vi "Shooter Controller.vi"(8 "error in":errorcluster) -> ()   [LabVIEW 2020]
doc: "This VI executes continuously carrying out the current operation and responding to updates or new operations. It will often contain the timing or control code that is difficult to place directly in TeleOp. This VI generally opens all sensors and motors and isolates the rest of the robot code from knowing how the operations are carried out."
uses:
  <vilib>/Rock Robotics/WPI/Framework/Completion Status.ctl
  Shooter Setpoints.ctl
  Shooter Operations.ctl
  <vilib>/Rock Robotics/WPI/SafetyOutput/WPI_SafetyOutputConfigMenu.ctl
  <vilib>/Rock Robotics/WPI/ThirdParty/REV Robotics/REVLib/Typedef/Spark MAX Motor Type.ctl
  <vilib>/Rock Robotics/WPI/ThirdParty/REV Robotics/REVLib/Typedef/Spark MAX Idle Mode.ctl
  <vilib>/Rock Robotics/Network Tables/NT Write Number.vi
panel:
  in  "Interactive Values":T1
  out "Current\nCmd":string
  in  "Buttons":cluster{"Execute Cmd":bool, "Abort Cmd":bool}
  out "Command Timing":cluster{"Start Time (ms)":u32, "Iterations":i32}
  out "Status":T3
  # "Tip: It may be helpful to observe inputs and sensor values.\nYou may also want to display tuning or debugging controls."
  # "Interactive Command: You may fill in the settings for a command\nand schedule it with the Execute button. You can observe and abort\nany command while fine tuning the code for the controller."
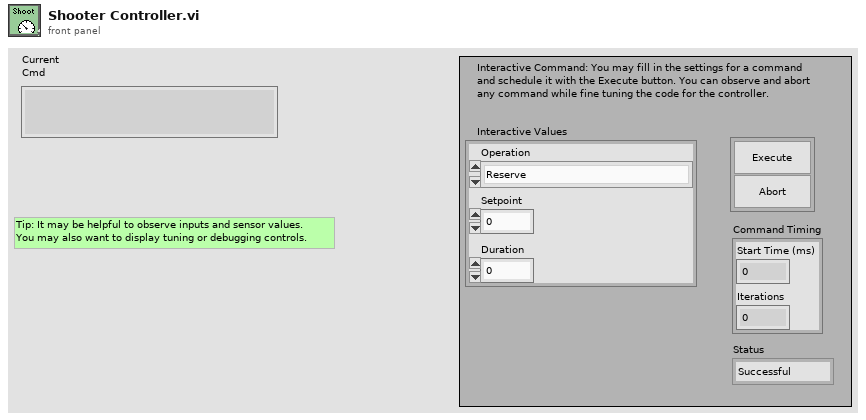
[diagram p1: front panel]
types:
  T1 = typedef "Shooter Setpoints.ctl" = cluster{"Operation":T2, "Setpoint":dbl, "Duration":dbl}
  T2 = typedef "Shooter Operations.ctl" = enum16{"Reserve", "Read Current", "Immediate", "For Time ", "Stop"}
  T3 = typedef "Completion Status.ctl" = enum16{"Successful", "Aborted", "Incomplete"}
  T4 = typedef "Spark MAX Idle Mode.ctl" = enum16{"Coast", "Brake"}
  T5 = typedef "Spark MAX Motor Type.ctl" = enum16{"Brushed", "Brushless"}
  T6 = typedef "WPI_SafetyOutputConfigMenu.ctl" = enum16{"Enable", "Disable"}
  T7 = typedef "WPI_MotorControlDeviceRef.ctl" = cluster{"DeviceStatus":errorcluster, "Type":T8, "PWM":cluster{"PWM Channel":T9, "DeadBand":T10}, "CAN":cluster{"Device Number":u8, "SetOutput VI Ref":variant, "GetOutput VI Ref":variant, "Enable VI Ref":variant, "Disable VI Ref":variant, "Data":variant}, "Invert":bool, "DIO PWM":cluster{"PWM \"Enable\" Channel":T9, "DIOChannel":T11, "PWM Rate":dbl}}
  T8 = typedef "WPI_MotorControlType.ctl" = enum16{"PWM", "CAN", "DIO PWM"}
  T9 = typedef "FPGA_DIOPWMChannel.ctl" = enum8{"PWM 0", "PWM 1", "PWM 2", "PWM 3", "PWM 4", "PWM 5", "PWM 6", "PWM 7", "PWM 8", "PWM 9", "PWM MXP 0", "PWM MXP 1", "PWM MXP 2", "PWM MXP 3", "PWM MXP 4", "PWM MXP 5", "PWM MXP 6", "PWM MXP 7", "PWM MXP 8", "PWM MXP 9", "Invalid"}
  T10 = typedef "WPI_PWMDeadband.ctl" = cluster{"Name":string, "maxPositivePwm":i32, "minPositivePwm":i32, "centerPwm":i32, "maxNegativePwm":i32, "minNegativePwm":i32, "angularRange":u16}
  T11 = typedef "FPGA_DIOChannel.ctl" = enum8{"DIO 0", "DIO 1", "DIO 2", "DIO 3", "DIO 4", "DIO 5", "DIO 6", "DIO 7", "DIO 8", "DIO 9", "DIO MXP 0", "DIO MXP 1", "DIO MXP 2", "DIO MXP 3", "DIO MXP 4", "DIO MXP 5", "DIO MXP 6", "DIO MXP 7", "DIO MXP 8", "DIO MXP 9", "DIO MXP 10", "DIO MXP 11", "DIO MXP 12", "DIO MXP 13", "DIO MXP 14", "DIO MXP 15", "SPI Port CS1", "SPI Port CS2", "SPI Port CS3", "SPI Port MISO", "SPI Port MOSI", "Invalid"}
  T12 = typedef "Command Status Info.ctl" = cluster{"Name":string, "Status":T3, "notifier out":T13}
  T13 = typedef "Completion Notifier.ctl" = refnum<notifier>
  T14 = cluster{"Current Command":T1, "Command Timing":cluster{"Start Time (ms)":u32, "Iterations":i32}, "Command Arguments":cluster{"Command Info":T12, "Description":string, "Default Command":T1, "queue out":refnum<queue>, "Subsystem Name":string}}
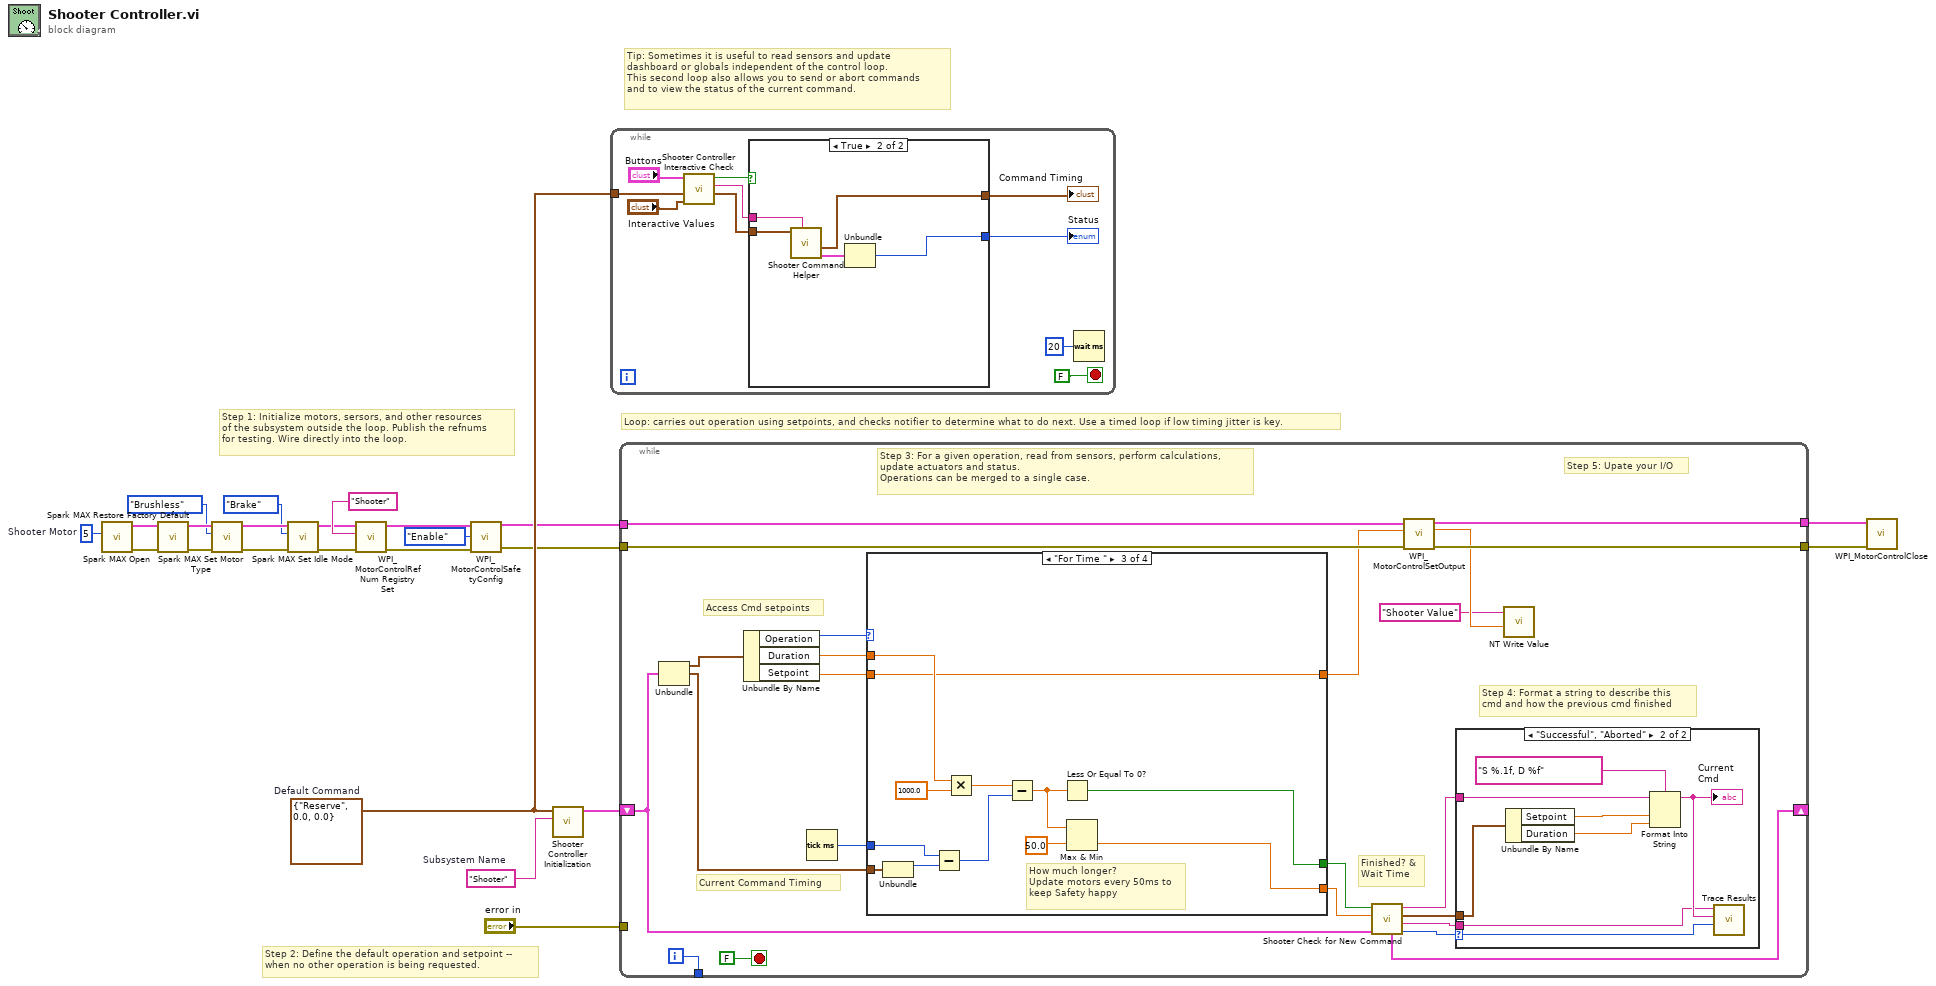
[diagram p0: block diagram]
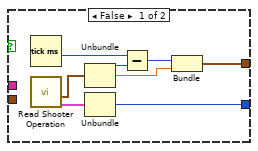
[diagram p2: hidden frame]
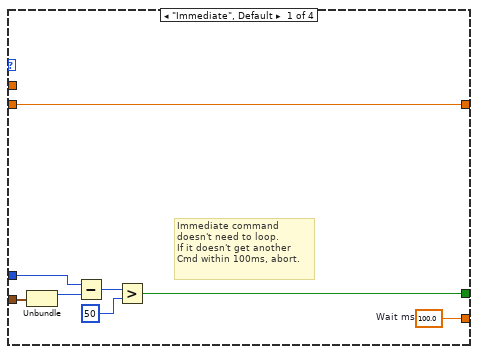
[diagram p4: hidden frame]
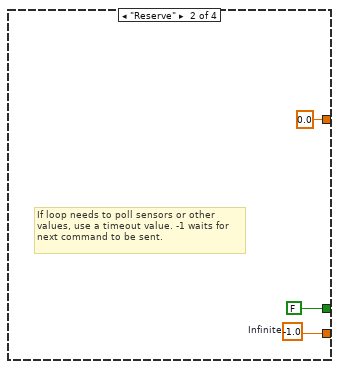
[diagram p5: hidden frame]
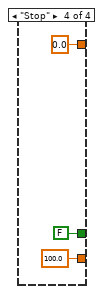
[diagram p6: hidden frame]
diagram:
  w1 = u8 5  # Shooter Motor
  w19 = T1 {"Operation"=enum."Reserve", "Setpoint"=0.0, "Duration"=0.0}  # Default Command
  w20 = "Shooter"  # Subsystem Name
  # "Tip: Sometimes it is useful to read sensors and update\ndashboard or globals independent of the control loop.\nThis second loop also allows you to send or abort commands\nand to view the status of the current command."
  # "Step 2: Define the default operation and setpoint --\nwhen no other operation is being requested."
  # "Step 1: Initialize motors, sersors, and other resources\nof the subsystem outside the loop. Publish the refnums\nfor testing. Wire directly into the loop."
  # "Loop: carries out operation using setpoints, and checks notifier to determine what to do next. Use a timed loop if low timing jitter is key."
  n1 = call <vilib>:"Spark MAX Open.vi"("Device Number"=w1) -> ("error out"=w18:errorcluster, "MotorControlDeviceRef"=w17:T7)  [unwired: 9 in]
  n2 = call <vilib>:"Spark MAX Restore Factory Default.vi"("error in"=w18, "MotorControlDeviceRef"=w17) -> ("error out"=w16:errorcluster, "MotorControlDeviceRef"=w15:T7)  [unwired: 8 in]
  n3 = call <vilib>:"Spark MAX Set Motor Type.vi"("error in (no error)"=w16, "Motor Type"=Spark_MAX_Motor_Type."Brushless", "MotorControlDevRef"=w15) -> ("error out"=w14:errorcluster, "MotorControlDeviceRef"=w13:T7)  [unwired: 7 in]
  n4 = call <vilib>:"Spark MAX Set Idle Mode.vi"("Idle Mode"=Spark_MAX_Idle_Mode."Brake", "MotorControlDeviceRef in"=w13) -> ("MotorControlDeviceRef out"=w7:T7)  [unwired: 8 in, 1 out]
  n5 = call <vilib>:"WPI_MotorControlRefNum Registry Set.vi"("error in (no error)"=w14, "refnum name"="Shooter", "MotorControlDevRef"=w7) -> ("error out"=w10:errorcluster, "MotorControlDevRef"=w12:T7)  [unwired: 7 in]
  n6 = call <vilib>:"WPI_MotorControlSafetyConfig.vi"("error in (no error)"=w10, "mode"=WPI_SafetyOutputConfigMenu."Enable", "MotorControlDevRef"=w12) -> ("error out"=w2:errorcluster, "MotorControlDevRef"=w5:T7)  [unwired: 7 in]
  n7 = call "Shooter Controller Initialization.vi"("Subsystem Name"=w20, "Default Command"=w19) -> ("Current Command"=w21:T14)  [unwired: 9 in]
  n8 = while {
    tunnel: w19 -> [w29]
    stop <- FALSE stop-if-true
    n9 = call "Shooter Controller Interactive Check.vi"("Interactive Command in"="Interactive Values", "Default Command"=w29, "Buttons"="Buttons") -> ("Interactive Command out"=w26:T1, "Trace String"=w27:string, "Schedule"=w28:bool)  [unwired: 6 in]
    n10 = case shown="True" w28 {
      tunnel: [w40 w45] -> w25
      tunnel: w26 -> [_ w43]
      tunnel: [w36 w41] -> w24
      tunnel: w27 -> [_ w44]
      frame False {
        n11 = Tick Count (ms)() -> (millisecond timer value=w35:u32)
        n12 = call "Read Shooter Operation.vi"() -> ("Command Info"=w33:T12, "SubSystem Data"=w34:T1)  [unwired: 9 in, 1 out]
        n13 = Unbundle(w34) -> ("Operation"=w39:T2, "Setpoint"=w37:dbl)  [unwired: 1 out]
        n14 = Unbundle(w33) -> ("Status"=w40:T3)  [unwired: 2 out]
        n15 = Subtract(x=w35, y=w39) -> (x-y=w38:u32)
        n16 = Bundle(w38, "Setpoint"=w37) -> (w36:cluster{u32, "Setpoint":dbl})  [unwired: 1 in]
      }
      frame True {
        n17 = call "Shooter Command Helper.vi"("Description"=w44, "SubSystem Data"=w43) -> ("Command Info Out"=w42:T12, "Command Timing"=w41:cluster{"Start Time (ms)":u32, "Iterations":i32})  [unwired: 7 in, 1 out]
        n18 = Unbundle(w42) -> ("Status"=w45:T3)  [unwired: 2 out]
      }
    }
    "Status" <- w25
    "Command Timing" <- w24
    n19 = Wait (ms)(milliseconds to wait=u32 20) -> ()  [unwired: 1 out]
  }
  n20 = while {
    shift-right: [w60] -> _
    shift-left: w21 -> [w53]
    tunnel: [w67] -> _
    tunnel: "error in" -> [_]
    tunnel: w5 -> [w52]
    tunnel: [w51] -> w4
    tunnel: [w50] -> w3
    tunnel: w2 -> [w49]
    i -> [w67]
    stop <- FALSE stop-if-true
    # "Step 5: Upate your I/O"
    # "Step 4: Format a string to describe this\ncmd and how the previous cmd finished"
    # "Current Command Timing"
    # "Access Cmd setpoints"
    # "Finished? &\nWait Time"
    # "Step 3: For a given operation, read from sensors, perform calculations,\nupdate actuators and status.\nOperations can be merged to a single case."
    n21 = Unbundle(w53) -> ("Current Command"=w66:T1, "Command Timing"=w62:cluster{"Start Time (ms)":u32, "Iterations":i32})  [unwired: 1 out]
    n22 = Unbundle By Name(w66) -> ("Operation"=w65:T2, "Duration"=w64:dbl, "Setpoint"=w61:dbl)
    n23 = Tick Count (ms)() -> (millisecond timer value=w63:u32)
    n24 = case shown="\"For Time \"" w65 {
      tunnel: [w84 w87 w90 100.0 ("Infinite")] -> w58
      tunnel: [w78 FALSE ("ignore previous (F)") w91 FALSE ("ignore previous (F)")] -> w59
      tunnel: w62 -> [w80 _ w92 _]
      tunnel: w64 -> [_ _ w89 _]
      tunnel: w63 -> [w79 _ w93 _]
      tunnel: w61 -> [w77 _ w88 _]
      tunnel: [w77 0.0 ("Setpoint") w88 0.0 ("Setpoint")] -> w46
      frame "Immediate", Default {
        w84 = 100.0  # Wait ms
        # "Immediate command\ndoesn't need to loop.\nIf it doesn't get another\nCmd within 100ms, abort."
        n25 = Unbundle(w80) -> ("Start Time (ms)"=w83:u32)  [unwired: 1 out]
        n26 = Subtract(x=w79, y=w83) -> (x-y=w82:u32)
        n27 = Greater?(x=w82, y=u8 50 ("Left Motor")) -> (0:w78:bool)
      }
      frame "Reserve" {
        w87 = -1.0  # Infinite
        # "If loop needs to poll sensors or other\nvalues, use a timeout value. -1 waits for\nnext command to be sent."
      }
      frame "For Time " {
        # "How much longer?\nUpdate motors every 50ms to\nkeep Safety happy"
        n28 = Unbundle(w92) -> ("Start Time (ms)"=w96:u32)  [unwired: 1 out]
        n29 = Subtract(x=w93, y=w96) -> (x-y=w99:u32)
        n30 = Multiply(x=w89, y=1000.0) -> (x*y=w98:dbl)
        n31 = Subtract(x=w98, y=w99) -> (x-y=w95:dbl)
        n32 = Less Or Equal To 0?(x=w95) -> (x <= 0?=w91:bool)
        n33 = Max & Min(x=w95, y=50.0) -> (min(x,y)=w90:dbl)  [unwired: 1 out]
      }
      frame "Stop" {
      }
    }
    n34 = call "Shooter Check for New Command.vi"("Current Command"=w53, "Wait time (ms)"=w58, "Finished?"=w59) -> ("Completion"=w54:T3, "Subsystem Name"=w55:string, "Current Command"=w56:T1, "Initial Trace String"=w57:string, "NextCommand"=w60:T14)  [unwired: 4 in]
    n35 = call <vilib>:"WPI_MotorControlSetOutput.vi"("error in (no error)"=w49, "Output"=w46, "MotorControlDevRef"=w52) -> ("error out"=w50:errorcluster, "Motor Output"=w48:dbl, "MotorControlDevRef"=w51:T7)  [unwired: 6 in]
    n36 = case shown="\"Successful\", \"Aborted\"" w54 {
      selector: w54 -> [_ w76]
      tunnel: w57 -> [_ w72]
      tunnel: w56 -> [_ w73]
      tunnel: w55 -> [_ w69]
      frame "Incomplete", Default {
        # "Continuing current command"
      }
      frame "Successful", "Aborted" {
        # "Report and setup for next command"
        n37 = Unbundle By Name(w73) -> ("Setpoint"=w75:dbl, "Duration"=w70:dbl)
        n38 = Format Into String(format string="S %.1f, D %f", initial string=w72, w75, w70) -> (resulting string=w71:string)  [unwired: 1 in, 1 out]
        "Current\nCmd" <- w71
        n39 = call <vilib>:"Trace Results.vi"("Status of previous command"=w76, "Description"=w71, "Subsystem"=w69) -> ()  [unwired: 9 in]
      }
    }
    n40 = call-poly <vilib>:"NT Write Value.vi"("Numeric"=w48, "Name"="Shooter Value") -> ()  [unwired: 9 in, 1 out]
  }
  n41 = call <vilib>:"WPI_MotorControlClose.vi"("error in"=w3, "MotorControlDevRef"=w4) -> ()  [unwired: 9 in, 1 out]
